vi "Class Roster Cluster--constant.vi"() -> (2 "Class Roster":T1)   [LabVIEW 2020]
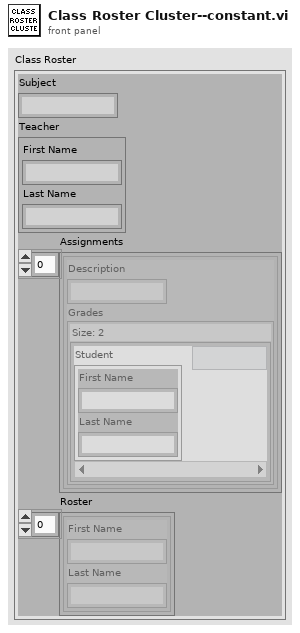
[diagram p1: front panel]
types:
  T1 = cluster{"Subject":string, "Teacher":cluster{"First Name":string, "Last Name":string}, "Assignments":cluster{"Description":string, "Grades":map{cluster{"First Name":string, "Last Name":string}, i32}}[], "Roster":cluster{"First Name":string, "Last Name":string}[]}
  T2 = cluster{"Description":string, "Grades":map{cluster{"First Name":string, "Last Name":string}, i32}}
  T3 = cluster{"First Name":string, "Last Name":string}[]
  T4 = map{cluster{"First Name":string, "Last Name":string}, i32}
  T5 = cluster{"Description":string, "Grades":map{cluster{"First Name":string, "Last Name":string}, i32}}[]
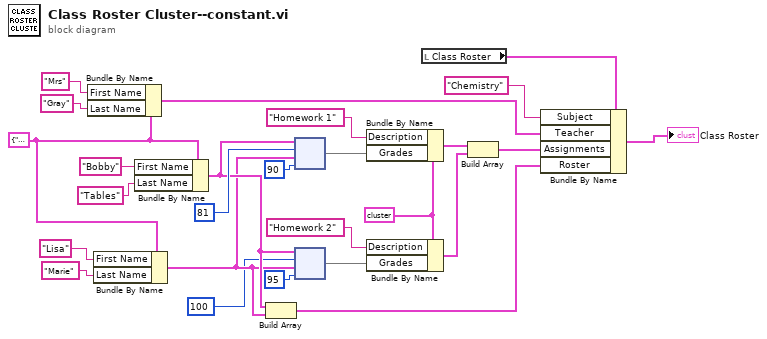
[diagram p0: block diagram]
diagram:
  w2 = T2 {"Description"="", "Grades"={}} ("Assignment")
  w23 = cluster{"First Name":string, "Last Name":string} {"First Name"="", "Last Name"=""} ("Student")
  n1 = Bundle By Name(cluster=w23, "First Name"="Mrs", "Last Name"="Gray") -> (w16:cluster{"First Name":string, "Last Name":string})
  n2 = Bundle By Name(cluster=w23, "First Name"="Lisa", "Last Name"="Marie") -> (w8:cluster{"First Name":string, "Last Name":string})
  n3 = Bundle By Name(cluster=w23, "First Name"="Bobby", "Last Name"="Tables") -> (w9:cluster{"First Name":string, "Last Name":string})
  n4 = Build Array(w9, w8) -> (w15:T3)
  n5 = node(w9, 81 ("value"), w8, 90 ("value")) -> (w12:T4)
  n6 = node(w9, 100 ("value"), w8, 95 ("value")) -> (w5:T4)
  n7 = Bundle By Name(cluster=w2, "Description"="Homework 1", "Grades"=w12) -> (w4:T2)
  n8 = Bundle By Name(cluster=w2, "Description"="Homework 2", "Grades"=w5) -> (w3:T2)
  n9 = local read "Class Roster"() -> (w26:T1)
  n10 = Build Array(w4, w3) -> (w1:T5)
  n11 = Bundle By Name(cluster=w26, "Subject"="Chemistry", "Teacher"=w16, "Assignments"=w1, "Roster"=w15) -> (→"Class Roster":T1)
